vi "1.1.Digital Blinking LED.vi"   [LabVIEW 2014]
doc: "This example shows how to set an Wemos D1 ESP8299 digital pin to an output, then toggle the voltage between low (0V) and high (3.3V) to drive an LED on and off."
uses:
  <vilib>/Aledyne-TSXperts/Arduino Compatible Compiler for LabVIEW/Code Generator/Arduino APIs/Digital/PinDirection.ctl
  <vilib>/Aledyne-TSXperts/Arduino Compatible Compiler for LabVIEW/Arduino Compatible Compiler for LabVIEW.lvlib
types:
  T1 = typedef "Arduino Compatible Compiler for LabVIEW.lvlib/PinDirection.ctl" = enum16{" INPUT", "OUTPUT", " INPUT_PULLUP"}
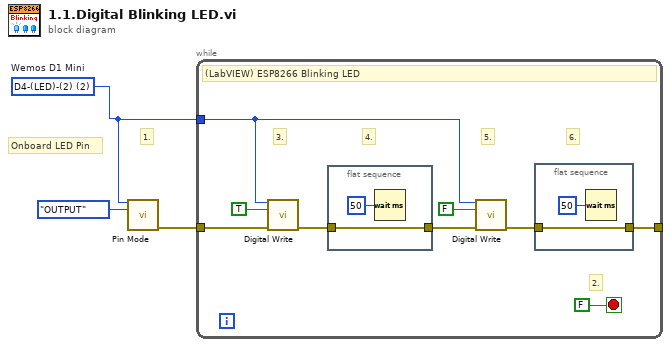
[diagram p0: block diagram]
diagram:
  w1 = u8 2 items=["D0-(16)"=16, "D1-SCL(5)"=5, "D2-SDA(4)"=4, "D3-(0)"=0, "D4-(LED)-(2)"=2, "D5-SCK(14)"=14, "D6-MISO(12)"=12, "D7-MOSI(13)"=13, "D8-SS(15)"=15, "TX(3)"=3, "RX(1)"=1, "ADC0,(17)"=17]  # Wemos D1 Mini
  # "Onboard LED Pin"
  # "1."
  n1 = call <vilib>:"Pin Mode.vi"("pin"=w1, "direction"=PinDirection."OUTPUT" ("Direction")) -> ("error out"=w3:errorcluster)  [unwired: 13 in]
  n2 = while {
    tunnel: w1 -> [w9]
    tunnel: w3 -> [w8]
    tunnel: [w10] -> _
    stop <- FALSE stop-if-true
    # "2."
    # "6."
    # "5."
    # "4."
    # "3."
    # "(LabVIEW) ESP8266 Blinking LED"
    n3 = call <vilib>:"Digital Write.vi"("pin"=w9, "state"=TRUE, "error in (no error)"=w8) -> ("error out"=w12:errorcluster)  [unwired: 12 in]
    n4 = flat-sequence {
      tunnel: [w15] -> w7
      tunnel: w12 -> [w15]
      frame #0 {
        n5 = Wait (ms)(milliseconds to wait=u32 50) -> ()  [unwired: 1 out]
      }
    }
    n6 = call <vilib>:"Digital Write.vi"("pin"=w9, "state"=FALSE, "error in (no error)"=w7) -> ("error out"=w11:errorcluster)  [unwired: 12 in]
    n7 = flat-sequence {
      tunnel: [w14] -> w10
      tunnel: w11 -> [w14]
      frame #0 {
        n8 = Wait (ms)(milliseconds to wait=u32 50) -> ()  [unwired: 1 out]
      }
    }
  }
